vi "To XML - With Method - Returns XML Entities.vi"() -> ()   [LabVIEW 2017, in "Cobertura.Tests.lvlib" / "Class.lvlib"]
uses:
  Class.lvlib
  <vilib>/xml/Close Reference(Node).vi
  Cobertura/Class/Class.lvclass
  <vilib>/xml/NI_XML.lvlib
  <resource>/objmgr/DOMUserDefRef.rc
  <vilib>/PNR/Transparent Assertions/Transparent Assertions/Transparent Assertions.lvlib
  Cobertura/Method/Method.lvclass
panel:
  out "error out":errorcluster
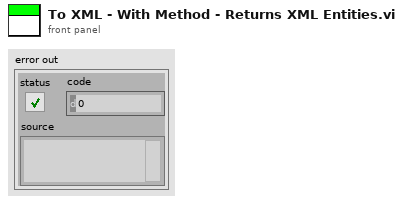
[diagram p1: front panel]
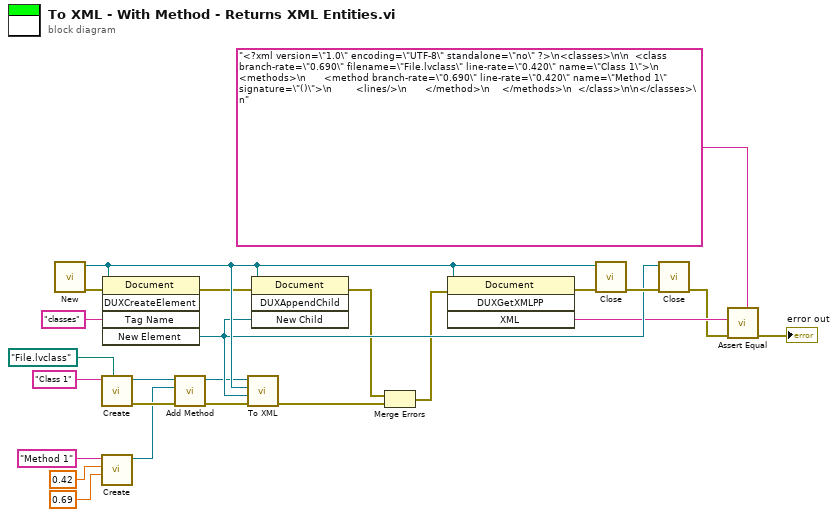
[diagram p0: block diagram]
diagram:
  n1 = call <vilib>:"New.vi"() -> ("error out"=w19:errorcluster, "DOM document out"=w21:refnum<k20>)  [unwired: 8 in]
  n2 = call "Create.vi"("Filename"=path "File.lvclass", "Name"="Class 1") -> ("error out"=w24:errorcluster, "Class"=w2:refnum<class "Class.lvclass">)  [unwired: 8 in]
  n3 = call "Create.vi"("Branch Rate"=0.69, "Line Rate"=0.42, "Name"="Method 1") -> ("Method"=w1:refnum<class "Method.lvclass">)  [unwired: 7 in, 1 out]
  n4 = invoke class="Document" method="DUXCreateElement"(reference=w21, error in=w19, "Tag Name"="classes") -> (error out=w20:errorcluster, "New Element"=w17:refnum<k20>)  [unwired: 2 in, 3 out]
  n5 = call "Add Method.vi"("error in (no error)"=w24, "Method"=w1, "Class in"=w2) -> ("error out"=w8:errorcluster, "Class out"=w7:refnum<class "Class.lvclass">)  [unwired: 7 in]
  n6 = call-dynamic "To XML.vi"("error in (no error)"=w8, "Parent"=w17, "Document"=w21, "Class in"=w7) -> ("error out"=w11:errorcluster)  [unwired: 7 in]
  n7 = invoke class="Document" method="DUXAppendChild"(reference=w21, error in=w20, "New Child"=w17) -> (error out=w13:errorcluster)  [unwired: 1 in, 3 out]
  n8 = Merge Errors(w13, w11) -> (w12:errorcluster)
  n9 = invoke class="Document" method="DUXGetXMLPP"(reference=w21, error in=w12) -> (error out=w22:errorcluster, "XML"=w16:string)  [unwired: 2 in, 2 out]
  n10 = call-poly <vilib>:"Close.vi"("error in (no error)"=w22, "node"=w21) -> ("error out"=w18:errorcluster)  [unwired: 7 in]
  n11 = call-poly <vilib>:"Close.vi"("error in (no error)"=w18, "node"=w17) -> ("error out"=w10:errorcluster)  [unwired: 7 in]
  n12 = call <vilib>:"Assert Equal.vi"("Expected"="<?xml version=\"1.0\" encoding=\"UTF-8\" standalone=\"no\" ?>\n<classes>\n\n  <class branch-rate=\"0.690\" filename=\"File.lvclass\" line-rate=\"0.420\" name=\"Class 1\">\n    <methods>\n      <method branch-rate=\"0.690\" line-rate=\"0.420\" name=\"Method 1\" signature=\"()\">\n        <lines/>\n      </method>\n    </methods>\n  </class>\n\n</classes>\n", "error in (no error)"=w10, "Actual"=w16) -> ("error out"=→"error out":errorcluster)  [unwired: 8 in]
